vi "UMLEditor UpdatesToolbuttons.vi"(1 "ClassTool":refnum<vi>, 2 "SequenceTool":refnum<vi>, 3 "UseCaseTool":refnum<vi>, 4 "StateTool":refnum<vi>, 5 "error in (no error)":errorcluster, 6 "Action(SelectSelect)":T1) -> (19 "error out":errorcluster)   [LabVIEW 2016]
doc: "Gets current diagram values"
uses:
  <resource>/Framework/Providers/Open_GDS/UML/UMLEditor/UMLEditor ToolButtonsAction.ctl
  <resource>/Framework/Providers/Open_GDS/UML/UMLEditor/UMLEditor ClassToolButtons.ctl
  <resource>/Framework/Providers/Open_GDS/UML/UMLEditor/UMLEditor SequenceToolButtons.ctl
  <resource>/Framework/Providers/Open_GDS/UML/UMLEditor/UMLEditor UseCaseToolButtons.ctl
  <resource>/Framework/Providers/Open_GDS/UML/UMLEditor/UMLEditor StateToolButtons.ctl
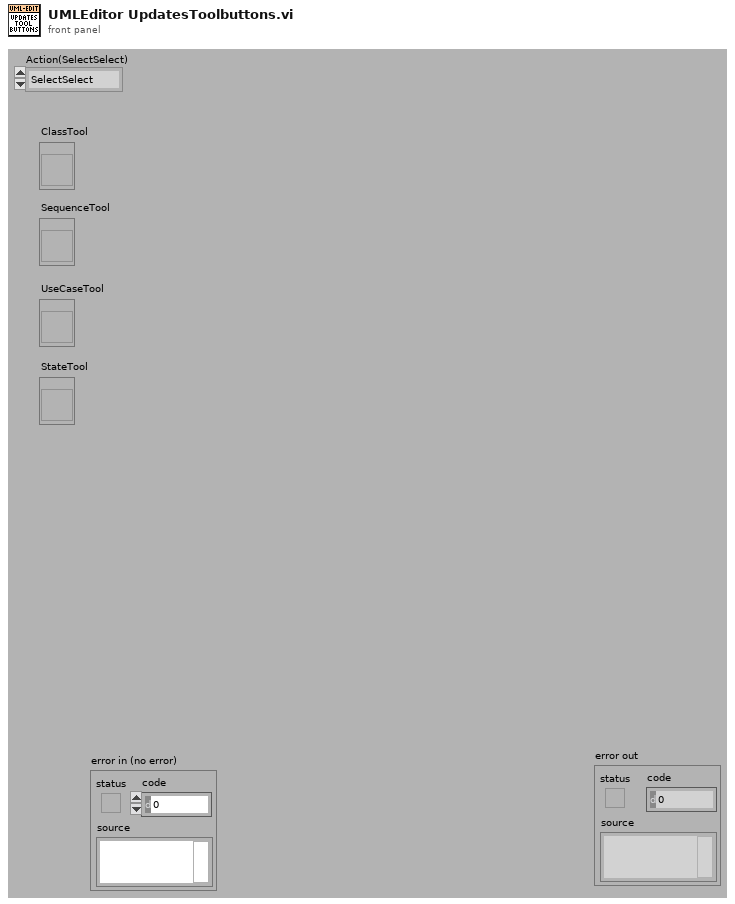
[diagram p1: front panel]
types:
  T1 = typedef "UMLEditor ToolButtonsAction.ctl" = enum16{"SelectSelect", "SetReferneces"}
  T2 = typedef "UMLEditor StateToolButtons.ctl" = cluster{"select":bool, "State":bool, "InitialState":bool, "FinalState":bool, "choice":bool, "StateTransation":bool, "note":bool, "noteConnect":bool}
  T3 = typedef "UMLEditor UseCaseToolButtons.ctl" = cluster{"select":bool, "System":bool, "Actor":bool, "UseCase":bool, "Association":bool, "Generalisation":bool, "Includes":bool, "Extends":bool, "Note":bool, "noteConnect":bool}
  T4 = typedef "UMLEditor SequenceToolButtons.ctl" = cluster{"select":bool, "Object":bool, "ActionBar":bool, "Call":bool, "note":bool, "noteConnect":bool}
  T5 = typedef "UMLEditor ClassToolButtons.ctl" = cluster{"select":bool, "class":bool, "interface":bool, "package":bool, "dependancy":bool, "inheritance":bool, "interfaceImp":bool, "association":bool, "aggregetion":bool, "compAggregetion":bool, "note":bool, "noteConnect":bool}
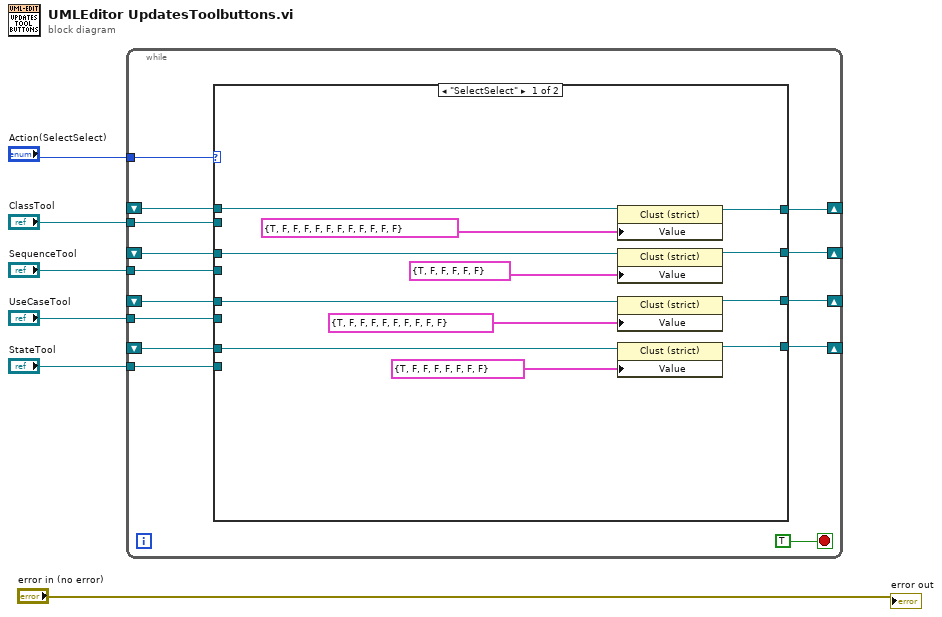
[diagram p0: block diagram]
diagram:
  n1 = while {
    tunnel: "Action(SelectSelect)" -> [w20]
    shift-right: [w17] -> _
    shift-left: _ -> [w18]
    shift-right: [w15] -> _
    shift-left: _ -> [w16]
    shift-right: [w12] -> _
    shift-left: _ -> [w14]
    shift-right: [w11] -> _
    shift-left: _ -> [w13]
    tunnel: "ClassTool" -> [w10]
    tunnel: "SequenceTool" -> [w9]
    tunnel: "UseCaseTool" -> [w8]
    tunnel: "StateTool" -> [w7]
    stop <- TRUE stop-if-true
    n2 = case shown="\"SelectSelect\"" w20 {
      tunnel: w18 -> [w32 _]
      tunnel: [w30 w36] -> w17
      tunnel: w16 -> [w29 _]
      tunnel: [w28 w35] -> w15
      tunnel: w14 -> [w26 _]
      tunnel: w13 -> [w25 _]
      tunnel: [w24 w34] -> w12
      tunnel: [w23 w33] -> w11
      tunnel: w10 -> [_ w36]
      tunnel: w9 -> [_ w35]
      tunnel: w8 -> [_ w34]
      tunnel: w7 -> [_ w33]
      frame "SelectSelect" {
        n3 = property class="Clust (strict)"(reference=w32, "Value"=T5 {"select"=TRUE, "class"=FALSE, "interface"=FALSE, "package"=FALSE, "dependancy"=FALSE, "inheritance"=FALSE, "interfaceImp"=FALSE, "association"=FALSE, "aggregetion"=FALSE, "compAggregetion"=FALSE, "note"=FALSE, "noteConnect"=FALSE} ("classDiagramTools")) -> (reference out=w30:refnum<vi>)  [unwired: 1 in, 1 out]
        n4 = property class="Clust (strict)"(reference=w29, "Value"=T4 {"select"=TRUE, "Object"=FALSE, "ActionBar"=FALSE, "Call"=FALSE, "note"=FALSE, "noteConnect"=FALSE} ("sequenceDiagramTools")) -> (reference out=w28:refnum<vi>)  [unwired: 1 in, 1 out]
        n5 = property class="Clust (strict)"(reference=w26, "Value"=T3 {"select"=TRUE, "System"=FALSE, "Actor"=FALSE, "UseCase"=FALSE, "Association"=FALSE, "Generalisation"=FALSE, "Includes"=FALSE, "Extends"=FALSE, "Note"=FALSE, "noteConnect"=FALSE} ("usecaseDiagramTools")) -> (reference out=w24:refnum<vi>)  [unwired: 1 in, 1 out]
        n6 = property class="Clust (strict)"(reference=w25, "Value"=T2 {"select"=TRUE, "State"=FALSE, "InitialState"=FALSE, "FinalState"=FALSE, "choice"=FALSE, "StateTransation"=FALSE, "note"=FALSE, "noteConnect"=FALSE} ("stateDiagramTools")) -> (reference out=w23:refnum<vi>)  [unwired: 1 in, 1 out]
      }
      frame "SetReferneces" {
      }
    }
  }
  "error out" <- "error in (no error)"
